vi "Select Platform.vi"(8 "error in (no error)":errorcluster, 10 "Platform":refnum<class "Platform.lvclass">, 11 "PlatformListPanel in":refnum<class "PlatformListPanel.lvclass">) -> (0 "error out":errorcluster, 3 "PlatformListPanel out":refnum<class "PlatformListPanel.lvclass">)   [LabVIEW 2020, in "PicoG-App.lvlib" / "PlatformListPanel.lvclass"]
uses:
  PlatformListPanel.lvclass
  PlatformListPanel.lvclass/PlatformListPanel.ctl
  PlatformArrayPanel/PlatformArrayPanel.lvclass
  <vilib>/IlluminatedG/IG OOPanel/OOPanel/ArrayManager/ArrayManager.lvclass
  Builds/picoG/ppl/PicoG-Core.lvlibp/PicoG-Processor/PicoG-Core/DeployPlatform/Platform.lvclass
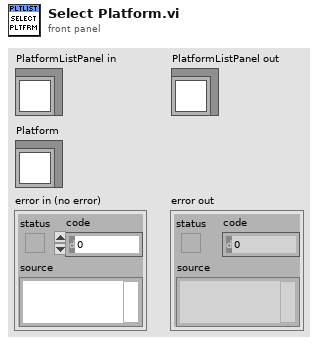
[diagram p1: front panel]
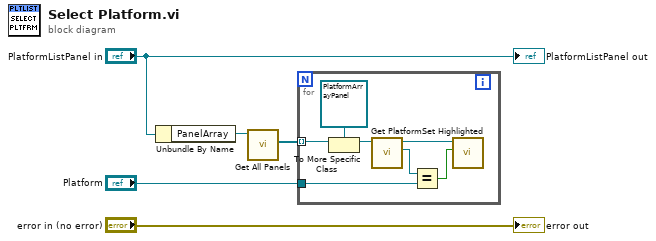
[diagram p0: block diagram]
diagram:
  n1 = Unbundle By Name("PlatformListPanel in") -> ("PanelArray"=w3:refnum<class "ArrayManager.lvclass">)
  n2 = call <vilib>:"Get All Panels.vi"("PanelArray in"=w3) -> ("Panels"=w2:refnum<class "ArrayPanel.lvclass">[])  [unwired: 8 in, 2 out]
  n3 = for {
    tunnel: w2 -> [w12] mode=indexing
    tunnel: "Platform" -> [w8]
    n4 = To More Specific Class(target class=refnum<class "PlatformArrayPanel.lvclass"> refnum ("PicoG-App.lvlib:PlatformArrayPanel.lvclass"), reference=w12) -> (specific class reference=w10:refnum<class "PlatformArrayPanel.lvclass">)  [unwired: 1 in, 1 out]
    n5 = call "Get Platform.vi"("PlatformArrayPanel in"=w10) -> ("Platform"=w7:refnum<class "Platform.lvclass">, "PlatformArrayPanel out"=w9:refnum<class "PlatformArrayPanel.lvclass">)  [unwired: 8 in, 1 out]
    n6 = Equal?(x=w7, y=w8) -> (x = y?=w6:bool)
    n7 = call "Set Highlighted.vi"("Highlighted"=w6, "PlatformArrayPanel in"=w9) -> ()  [unwired: 8 in, 2 out]
  }
  "error out" <- "error in (no error)"
  "PlatformListPanel out" <- "PlatformListPanel in"
